vi "InitCAN_ATII.vi"(1 "Config":refnum<vi>) -> (0 "Sts":bool)   [LabVIEW 2017]
uses:
  PCAN_Driver/ControlCAN.llb/Return Val.ctl
  PCAN_Driver/ControlCAN.lvlib
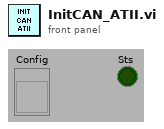
[diagram p1: front panel]
types:
  T1 = typedef "ControlCAN.lvlib/Return Val.ctl" = i32
  T2 = typedef "ControlCAN.lvlib/DevType.ctl" = u32
  T3 = typedef "ControlCAN.lvlib/CAN Channel.ctl" = u32
  T4 = typedef "ControlCAN.lvlib/VCI_INIT_CONFIG.ctl" = cluster{"AccCode":u32, "AccMask":u32, "InitFlag":T5, "Fliter":T6, "Timing0":u8, "Timing1":u8, "Mode":T7}
  T5 = typedef "ControlCAN.lvlib/InitFlag.ctl" = u32
  T6 = typedef "ControlCAN.lvlib/Fliter.ctl" = u8
  T7 = typedef "ControlCAN.lvlib/Mode.ctl" = u8
  T8 = cluster{"DevType":T2, "DevIndex":u32, "CanIndex":T3, "VCI_INIT_CONFIG":T4}
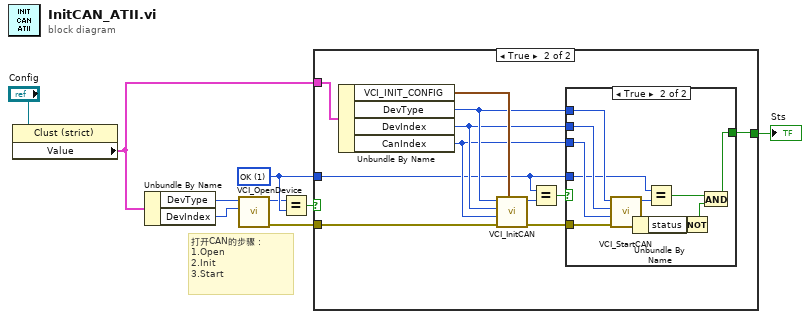
[diagram p0: block diagram]
diagram:
  w7 = T1 1 items=["OK"=1, "ERROR1"=0, "ERROR2"=-1] ("y")
  # "打开CAN的步骤：\n1.Open\n2.Init\n3.Start"
  n1 = property class="Clust (strict)"(reference="Config") -> ("Value"=w8:T8)  [unwired: 1 in, 2 out]
  n2 = Unbundle By Name(w8) -> ("DevType"=w2:T2, "DevIndex"=w3:u32)
  n3 = call "VCI_OpenDevice.vi"("DevIndex"=w3, "DevType"=w2) -> ("error out"=w6:errorcluster, "Return Val"=w4:T1)  [unwired: 2 in, 6 out]
  n4 = Equal?(x=w4, y=w7) -> (x = y?=w5:bool)
  n5 = case shown="True" w5 {
    tunnel: w6 -> [_ w20]
    tunnel: w8 -> [_ w19]
    tunnel: w7 -> [_ w11]
    tunnel: [_ w10] -> w9
    frame False {
    }
    frame True {
      n6 = Unbundle By Name(w19) -> ("VCI_INIT_CONFIG"=w18:T4, "DevType"=w14:T2, "DevIndex"=w13:u32, "CanIndex"=w12:T3)
      n7 = call "VCI_InitCAN.vi"("VCI_INIT_CONFIG"=w18, "error in (no error)"=w20, "CANIndex"=w12, "DevIndex"=w13, "DevType"=w14) -> ("error out"=w15:errorcluster, "Return Val"=w17:T1)  [unwired: 5 out]
      n8 = Equal?(x=w11, y=w17) -> (x = y?=w16:bool)
      n9 = case shown="True" w16 {
        tunnel: w15 -> [_ w31]
        tunnel: w14 -> [_ w30]
        tunnel: w13 -> [_ w29]
        tunnel: w12 -> [_ w28]
        tunnel: w11 -> [_ w26]
        tunnel: [_ w22] -> w10
        frame False {
        }
        frame True {
          n10 = call "VCI_StartCAN.vi"("error in (no error)"=w31, "CANIndex"=w28, "DevIndex"=w29, "DevType"=w30) -> ("error out"=w24:errorcluster, "Return Val"=w27:T1)  [unwired: 6 out]
          n11 = Unbundle By Name(w24) -> ("status"=w21:bool)
          n12 = Equal?(x=w26, y=w27) -> (x = y?=w25:bool)
          n13 = Not(x=w21) -> (.not. x?=w23:bool)
          n14 = And(x=w25, y=w23) -> (x .and. y?=w22:bool)
        }
      }
    }
  }
  "Sts" <- w9
